vi "setUserEvent.vi"(8 "error in (no error)":errorcluster, 11 "GeneralDisplay in":refnum<class "GeneralDisplay.lvclass">) -> (0 "error out":errorcluster, 3 "GeneralDisplay out":refnum<class "GeneralDisplay.lvclass">)   [LabVIEW 2017, in "GeneralDisplay.lvclass"]
uses:
  GeneralDisplay.lvclass
  Observer/Observer.lvclass
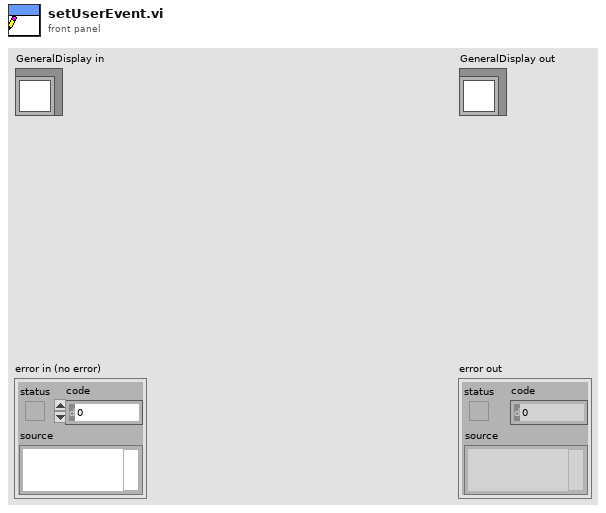
[diagram p1: front panel]
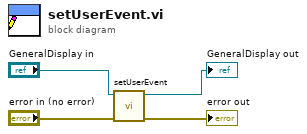
[diagram p0: block diagram]
diagram:
  n1 = call-parent "setUserEvent.vi"("error in (no error)"="error in (no error)", "Observer in"="GeneralDisplay in") -> ("error out"=→"error out":errorcluster, "Observer out"=→"GeneralDisplay out":refnum<class "GeneralDisplay.lvclass">)  [unwired: 8 in]
